vi "main(Test DQMH modules).vi"() -> ()   [LabVIEW 2018, in "Application.lvlib"] (continued)
        n2834 = Bundle By Name(cluster=w6304, "command"="Apps.WaitForEvent", "command data"=w6299) -> (w6303:T11)
        n2835 = Bundle By Name(cluster=w6304, "command"="MEAS.DMM dual read") -> (w6319:T11)
        n2836 = Bundle By Name(cluster=w6304, "command"="Apps.UI Update 1") -> (w6305:T11)
        n2837 = Build Array(w6319, w6318, w6303, w6305) -> (w6316:T11[])
        n2838 = Build Array (concatenate)(w6317, w6316) -> (w6315:T11[])
        n2839 = for {
          tunnel: w6315 -> [w6353] mode=indexing
          tunnel: w6310 -> [w6354]
          tunnel: [w6350] -> w6313 mode=indexing
          n2840 = Unbundle By Name(w6353) -> ("command"=w6352:string, "command data"=w6351:variant)
          n2841 = call "App enquece.vi"("command data"=w6351, "command"=w6352, "queue in"=w6354) -> ("error out"=w6350:errorcluster)  [unwired: 7 in, 1 out]
        }
        n2842 = Merge Errors(w6314, w6313) -> (w6312:errorcluster)
      }
      frame "Test DRV 6A" {
        w6361 = T11 {"command"="", "command data"=variant} ("element")
        w6355 = 6 ("DUT index(0-59)")
        w6387 = T11 {"command"="", "command data"=variant} ("element")
        n2843 = disable-structure shown="LOGGING==TRUE" {
          disable-tunnel: w6365 -> [w6403 _]
          frame condition #0 (active) {
            n2844 = Empty String/Path?(string/path=w6403) -> (empty?=w6406:bool)
            n2845 = Select(t="Quece timeout", s=w6406, f=w6403) -> (s? t:f=w6402:string)
            n2846 = call "string log (SubVI).vi"("Enum"=enum16{"Init", "Log", "Read"}."Log", "state Name"=w6402) -> ()  [unwired: 8 in, 2 out]
          }
          frame condition #1 {
          }
        }
        n2847 = Flush Queue(queue=w6366) -> (queue out=w6367:refnum<queue>)  [unwired: 1 in, 2 out]
        n2848 = Decrement(x=w6355) -> (x-1=w6359:i32)
        n2849 = Index Array(array=w6356, index=w6359) -> (element=w6357:refnum<vi>)
        n2850 = property class="ColBox"(reference=w6357, "Value"=u32 10000536 ("DRV 1")) -> ()  [unwired: 1 in, 2 out]
        n2851 = To Variant(anything=bool[] [FALSE, FALSE, FALSE, FALSE, FALSE, TRUE]) -> (Variant=w6384:variant)
        n2852 = To Variant(anything=T6."demux1_10_channel1" ("demux1_10(x6)_encode")) -> (Variant=w6388:variant)
        n2853 = To Variant(anything=T4."mux6_1_channel5_3" ("mux6_1(3wires)_encode")) -> (Variant=w6392:variant)
        n2854 = To Variant(anything=T5."mux10_1_channel1" ("mux10_1(x6)_encode")) -> (Variant=w6394:variant)
        n2855 = Bundle By Name(cluster=w6387, "command"="MEAS.mux10-1", "command data"=w6394) -> (w6382:T11)
        n2856 = Bundle By Name(cluster=w6387, "command"="MEAS.mux6_1", "command data"=w6392) -> (w6381:T11)
        n2857 = Bundle By Name(cluster=w6387, "command"="MEAS.demux1-10", "command data"=w6388) -> (w6380:T11)
        n2858 = Bundle By Name(cluster=w6387, "command"="MEAS.eMIC", "command data"=w6384) -> (w6379:T11)
        n2859 = Bundle By Name(cluster=w6387, "command"="MEAS.AllRelaysOFF") -> (w6383:T11)
        n2860 = Build Array(w6383, w6382, w6381, w6380, w6379) -> (w6374:T11[])
        n2861 = Bundle By Name(cluster=w6361, "command"="MEAS.requestAC", "command data"=w6355) -> (w6375:T11)
        n2862 = Bundle By Name(cluster=w6361, "command"="Apps.WaitForEvent", "command data"=w6355) -> (w6360:T11)
        n2863 = Bundle By Name(cluster=w6361, "command"="MEAS.DMM dual read") -> (w6376:T11)
        n2864 = Bundle By Name(cluster=w6361, "command"="Apps.UI Update 1") -> (w6362:T11)
        n2865 = Build Array(w6376, w6375, w6360, w6362) -> (w6373:T11[])
        n2866 = Build Array (concatenate)(w6374, w6373) -> (w6372:T11[])
        n2867 = for {
          tunnel: w6372 -> [w6410] mode=indexing
          tunnel: w6367 -> [w6411]
          tunnel: [w6407] -> w6370 mode=indexing
          n2868 = Unbundle By Name(w6410) -> ("command"=w6409:string, "command data"=w6408:variant)
          n2869 = call "App enquece.vi"("command data"=w6408, "command"=w6409, "queue in"=w6411) -> ("error out"=w6407:errorcluster)  [unwired: 7 in, 1 out]
        }
        n2870 = Merge Errors(w6371, w6370) -> (w6369:errorcluster)
      }
      frame "Test DRV 7A" {
        w6418 = T11 {"command"="", "command data"=variant} ("element")
        w6412 = 7 ("DUT index(0-59)")
        w6444 = T11 {"command"="", "command data"=variant} ("element")
        n2871 = disable-structure shown="LOGGING==TRUE" {
          disable-tunnel: w6422 -> [w6460 _]
          frame condition #0 (active) {
            n2872 = Empty String/Path?(string/path=w6460) -> (empty?=w6463:bool)
            n2873 = Select(t="Quece timeout", s=w6463, f=w6460) -> (s? t:f=w6459:string)
            n2874 = call "string log (SubVI).vi"("Enum"=enum16{"Init", "Log", "Read"}."Log", "state Name"=w6459) -> ()  [unwired: 8 in, 2 out]
          }
          frame condition #1 {
          }
        }
        n2875 = Flush Queue(queue=w6423) -> (queue out=w6424:refnum<queue>)  [unwired: 1 in, 2 out]
        n2876 = Decrement(x=w6412) -> (x-1=w6416:i32)
        n2877 = Index Array(array=w6413, index=w6416) -> (element=w6414:refnum<vi>)
        n2878 = property class="ColBox"(reference=w6414, "Value"=u32 10000536 ("DRV 1")) -> ()  [unwired: 1 in, 2 out]
        n2879 = To Variant(anything=bool[] [TRUE, FALSE, FALSE, FALSE, FALSE, FALSE]) -> (Variant=w6441:variant)
        n2880 = To Variant(anything=T6."demux1_10_channel2" ("demux1_10(x6)_encode")) -> (Variant=w6445:variant)
        n2881 = To Variant(anything=T4."mux6_1_channel1_3" ("mux6_1(3wires)_encode")) -> (Variant=w6449:variant)
        n2882 = To Variant(anything=T5."mux10_1_channel2" ("mux10_1(x6)_encode")) -> (Variant=w6451:variant)
        n2883 = Bundle By Name(cluster=w6444, "command"="MEAS.mux10-1", "command data"=w6451) -> (w6439:T11)
        n2884 = Bundle By Name(cluster=w6444, "command"="MEAS.mux6_1", "command data"=w6449) -> (w6438:T11)
        n2885 = Bundle By Name(cluster=w6444, "command"="MEAS.demux1-10", "command data"=w6445) -> (w6437:T11)
        n2886 = Bundle By Name(cluster=w6444, "command"="MEAS.eMIC", "command data"=w6441) -> (w6436:T11)
        n2887 = Bundle By Name(cluster=w6444, "command"="MEAS.AllRelaysOFF") -> (w6440:T11)
        n2888 = Build Array(w6440, w6439, w6438, w6437, w6436) -> (w6431:T11[])
        n2889 = Bundle By Name(cluster=w6418, "command"="MEAS.requestAC", "command data"=w6412) -> (w6432:T11)
        n2890 = Bundle By Name(cluster=w6418, "command"="Apps.WaitForEvent", "command data"=w6412) -> (w6417:T11)
        n2891 = Bundle By Name(cluster=w6418, "command"="MEAS.DMM dual read") -> (w6433:T11)
        n2892 = Bundle By Name(cluster=w6418, "command"="Apps.UI Update 1") -> (w6419:T11)
        n2893 = Build Array(w6433, w6432, w6417, w6419) -> (w6430:T11[])
        n2894 = Build Array (concatenate)(w6431, w6430) -> (w6429:T11[])
        n2895 = for {
          tunnel: w6429 -> [w6467] mode=indexing
          tunnel: w6424 -> [w6468]
          tunnel: [w6464] -> w6427 mode=indexing
          n2896 = Unbundle By Name(w6467) -> ("command"=w6466:string, "command data"=w6465:variant)
          n2897 = call "App enquece.vi"("command data"=w6465, "command"=w6466, "queue in"=w6468) -> ("error out"=w6464:errorcluster)  [unwired: 7 in, 1 out]
        }
        n2898 = Merge Errors(w6428, w6427) -> (w6426:errorcluster)
      }
      frame "Test DRV 8A" {
        w6475 = T11 {"command"="", "command data"=variant} ("element")
        w6469 = 8 ("DUT index(0-59)")
        w6501 = T11 {"command"="", "command data"=variant} ("element")
        n2899 = disable-structure shown="LOGGING==TRUE" {
          disable-tunnel: w6479 -> [w6517 _]
          frame condition #0 (active) {
            n2900 = Empty String/Path?(string/path=w6517) -> (empty?=w6520:bool)
            n2901 = Select(t="Quece timeout", s=w6520, f=w6517) -> (s? t:f=w6516:string)
            n2902 = call "string log (SubVI).vi"("Enum"=enum16{"Init", "Log", "Read"}."Log", "state Name"=w6516) -> ()  [unwired: 8 in, 2 out]
          }
          frame condition #1 {
          }
        }
        n2903 = Flush Queue(queue=w6480) -> (queue out=w6481:refnum<queue>)  [unwired: 1 in, 2 out]
        n2904 = Decrement(x=w6469) -> (x-1=w6473:i32)
        n2905 = Index Array(array=w6470, index=w6473) -> (element=w6471:refnum<vi>)
        n2906 = property class="ColBox"(reference=w6471, "Value"=u32 10000536 ("DRV 1")) -> ()  [unwired: 1 in, 2 out]
        n2907 = To Variant(anything=bool[] [FALSE, TRUE, FALSE, FALSE, FALSE, FALSE]) -> (Variant=w6498:variant)
        n2908 = To Variant(anything=T6."demux1_10_channel2" ("demux1_10(x6)_encode")) -> (Variant=w6502:variant)
        n2909 = To Variant(anything=T4."mux6_1_channel2_3" ("mux6_1(3wires)_encode")) -> (Variant=w6506:variant)
        n2910 = To Variant(anything=T5."mux10_1_channel2" ("mux10_1(x6)_encode")) -> (Variant=w6508:variant)
        n2911 = Bundle By Name(cluster=w6501, "command"="MEAS.mux10-1", "command data"=w6508) -> (w6496:T11)
        n2912 = Bundle By Name(cluster=w6501, "command"="MEAS.mux6_1", "command data"=w6506) -> (w6495:T11)
        n2913 = Bundle By Name(cluster=w6501, "command"="MEAS.demux1-10", "command data"=w6502) -> (w6494:T11)
        n2914 = Bundle By Name(cluster=w6501, "command"="MEAS.eMIC", "command data"=w6498) -> (w6493:T11)
        n2915 = Bundle By Name(cluster=w6501, "command"="MEAS.AllRelaysOFF") -> (w6497:T11)
        n2916 = Build Array(w6497, w6496, w6495, w6494, w6493) -> (w6488:T11[])
        n2917 = Bundle By Name(cluster=w6475, "command"="MEAS.requestAC", "command data"=w6469) -> (w6489:T11)
        n2918 = Bundle By Name(cluster=w6475, "command"="Apps.WaitForEvent", "command data"=w6469) -> (w6474:T11)
        n2919 = Bundle By Name(cluster=w6475, "command"="MEAS.DMM dual read") -> (w6490:T11)
        n2920 = Bundle By Name(cluster=w6475, "command"="Apps.UI Update 1") -> (w6476:T11)
        n2921 = Build Array(w6490, w6489, w6474, w6476) -> (w6487:T11[])
        n2922 = Build Array (concatenate)(w6488, w6487) -> (w6486:T11[])
        n2923 = for {
          tunnel: w6486 -> [w6524] mode=indexing
          tunnel: w6481 -> [w6525]
          tunnel: [w6521] -> w6484 mode=indexing
          n2924 = Unbundle By Name(w6524) -> ("command"=w6523:string, "command data"=w6522:variant)
          n2925 = call "App enquece.vi"("command data"=w6522, "command"=w6523, "queue in"=w6525) -> ("error out"=w6521:errorcluster)  [unwired: 7 in, 1 out]
        }
        n2926 = Merge Errors(w6485, w6484) -> (w6483:errorcluster)
      }
      frame "Test DRV 9A" {
        w6532 = T11 {"command"="", "command data"=variant} ("element")
        w6526 = 9 ("DUT index(0-59)")
        w6558 = T11 {"command"="", "command data"=variant} ("element")
        n2927 = disable-structure shown="LOGGING==TRUE" {
          disable-tunnel: w6536 -> [w6574 _]
          frame condition #0 (active) {
            n2928 = Empty String/Path?(string/path=w6574) -> (empty?=w6577:bool)
            n2929 = Select(t="Quece timeout", s=w6577, f=w6574) -> (s? t:f=w6573:string)
            n2930 = call "string log (SubVI).vi"("Enum"=enum16{"Init", "Log", "Read"}."Log", "state Name"=w6573) -> ()  [unwired: 8 in, 2 out]
          }
          frame condition #1 {
          }
        }
        n2931 = Flush Queue(queue=w6537) -> (queue out=w6538:refnum<queue>)  [unwired: 1 in, 2 out]
        n2932 = Decrement(x=w6526) -> (x-1=w6530:i32)
        n2933 = Index Array(array=w6527, index=w6530) -> (element=w6528:refnum<vi>)
        n2934 = property class="ColBox"(reference=w6528, "Value"=u32 10000536 ("DRV 1")) -> ()  [unwired: 1 in, 2 out]
        n2935 = To Variant(anything=bool[] [FALSE, FALSE, TRUE, FALSE, FALSE, FALSE]) -> (Variant=w6555:variant)
        n2936 = To Variant(anything=T6."demux1_10_channel2" ("demux1_10(x6)_encode")) -> (Variant=w6559:variant)
        n2937 = To Variant(anything=T4."mux6_1_channel3_3" ("mux6_1(3wires)_encode")) -> (Variant=w6563:variant)
        n2938 = To Variant(anything=T5."mux10_1_channel2" ("mux10_1(x6)_encode")) -> (Variant=w6565:variant)
        n2939 = Bundle By Name(cluster=w6558, "command"="MEAS.mux10-1", "command data"=w6565) -> (w6553:T11)
        n2940 = Bundle By Name(cluster=w6558, "command"="MEAS.mux6_1", "command data"=w6563) -> (w6552:T11)
        n2941 = Bundle By Name(cluster=w6558, "command"="MEAS.demux1-10", "command data"=w6559) -> (w6551:T11)
        n2942 = Bundle By Name(cluster=w6558, "command"="MEAS.eMIC", "command data"=w6555) -> (w6550:T11)
        n2943 = Bundle By Name(cluster=w6558, "command"="MEAS.AllRelaysOFF") -> (w6554:T11)
        n2944 = Build Array(w6554, w6553, w6552, w6551, w6550) -> (w6545:T11[])
        n2945 = Bundle By Name(cluster=w6532, "command"="MEAS.requestAC", "command data"=w6526) -> (w6546:T11)
        n2946 = Bundle By Name(cluster=w6532, "command"="Apps.WaitForEvent", "command data"=w6526) -> (w6531:T11)
        n2947 = Bundle By Name(cluster=w6532, "command"="MEAS.DMM dual read") -> (w6547:T11)
        n2948 = Bundle By Name(cluster=w6532, "command"="Apps.UI Update 1") -> (w6533:T11)
        n2949 = Build Array(w6547, w6546, w6531, w6533) -> (w6544:T11[])
        n2950 = Build Array (concatenate)(w6545, w6544) -> (w6543:T11[])
        n2951 = for {
          tunnel: w6543 -> [w6581] mode=indexing
          tunnel: w6538 -> [w6582]
          tunnel: [w6578] -> w6541 mode=indexing
          n2952 = Unbundle By Name(w6581) -> ("command"=w6580:string, "command data"=w6579:variant)
          n2953 = call "App enquece.vi"("command data"=w6579, "command"=w6580, "queue in"=w6582) -> ("error out"=w6578:errorcluster)  [unwired: 7 in, 1 out]
        }
        n2954 = Merge Errors(w6542, w6541) -> (w6540:errorcluster)
      }
      frame "Test DRV 10A" {
        w6589 = T11 {"command"="", "command data"=variant} ("element")
        w6583 = 10 ("DUT index(0-59)")
        w6615 = T11 {"command"="", "command data"=variant} ("element")
        n2955 = disable-structure shown="LOGGING==TRUE" {
          disable-tunnel: w6593 -> [w6631 _]
          frame condition #0 (active) {
            n2956 = Empty String/Path?(string/path=w6631) -> (empty?=w6634:bool)
            n2957 = Select(t="Quece timeout", s=w6634, f=w6631) -> (s? t:f=w6630:string)
            n2958 = call "string log (SubVI).vi"("Enum"=enum16{"Init", "Log", "Read"}."Log", "state Name"=w6630) -> ()  [unwired: 8 in, 2 out]
          }
          frame condition #1 {
          }
        }
        n2959 = Flush Queue(queue=w6594) -> (queue out=w6595:refnum<queue>)  [unwired: 1 in, 2 out]
        n2960 = Decrement(x=w6583) -> (x-1=w6587:i32)
        n2961 = Index Array(array=w6584, index=w6587) -> (element=w6585:refnum<vi>)
        n2962 = property class="ColBox"(reference=w6585, "Value"=u32 10000536 ("DRV 1")) -> ()  [unwired: 1 in, 2 out]
        n2963 = To Variant(anything=bool[] [FALSE, FALSE, FALSE, TRUE, FALSE, FALSE]) -> (Variant=w6612:variant)
        n2964 = To Variant(anything=T6."demux1_10_channel2" ("demux1_10(x6)_encode")) -> (Variant=w6616:variant)
        n2965 = To Variant(anything=T4."mux6_1_channel4_3" ("mux6_1(3wires)_encode")) -> (Variant=w6620:variant)
        n2966 = To Variant(anything=T5."mux10_1_channel2" ("mux10_1(x6)_encode")) -> (Variant=w6622:variant)
        n2967 = Bundle By Name(cluster=w6615, "command"="MEAS.mux10-1", "command data"=w6622) -> (w6610:T11)
        n2968 = Bundle By Name(cluster=w6615, "command"="MEAS.mux6_1", "command data"=w6620) -> (w6609:T11)
        n2969 = Bundle By Name(cluster=w6615, "command"="MEAS.demux1-10", "command data"=w6616) -> (w6608:T11)
        n2970 = Bundle By Name(cluster=w6615, "command"="MEAS.eMIC", "command data"=w6612) -> (w6607:T11)
        n2971 = Bundle By Name(cluster=w6615, "command"="MEAS.AllRelaysOFF") -> (w6611:T11)
        n2972 = Build Array(w6611, w6610, w6609, w6608, w6607) -> (w6602:T11[])
        n2973 = Bundle By Name(cluster=w6589, "command"="MEAS.requestAC", "command data"=w6583) -> (w6603:T11)
        n2974 = Bundle By Name(cluster=w6589, "command"="Apps.WaitForEvent", "command data"=w6583) -> (w6588:T11)
        n2975 = Bundle By Name(cluster=w6589, "command"="MEAS.DMM dual read") -> (w6604:T11)
        n2976 = Bundle By Name(cluster=w6589, "command"="Apps.UI Update 1") -> (w6590:T11)
        n2977 = Build Array(w6604, w6603, w6588, w6590) -> (w6601:T11[])
        n2978 = Build Array (concatenate)(w6602, w6601) -> (w6600:T11[])
        n2979 = for {
          tunnel: w6600 -> [w6638] mode=indexing
          tunnel: w6595 -> [w6639]
          tunnel: [w6635] -> w6598 mode=indexing
          n2980 = Unbundle By Name(w6638) -> ("command"=w6637:string, "command data"=w6636:variant)
          n2981 = call "App enquece.vi"("command data"=w6636, "command"=w6637, "queue in"=w6639) -> ("error out"=w6635:errorcluster)  [unwired: 7 in, 1 out]
        }
        n2982 = Merge Errors(w6599, w6598) -> (w6597:errorcluster)
      }
      frame "Test DRV 11A" {
        w6646 = T11 {"command"="", "command data"=variant} ("element")
        w6640 = 11 ("DUT index(0-59)")
        w6672 = T11 {"command"="", "command data"=variant} ("element")
        n2983 = disable-structure shown="LOGGING==TRUE" {
          disable-tunnel: w6650 -> [w6688 _]
          frame condition #0 (active) {
            n2984 = Empty String/Path?(string/path=w6688) -> (empty?=w6691:bool)
            n2985 = Select(t="Quece timeout", s=w6691, f=w6688) -> (s? t:f=w6687:string)
            n2986 = call "string log (SubVI).vi"("Enum"=enum16{"Init", "Log", "Read"}."Log", "state Name"=w6687) -> ()  [unwired: 8 in, 2 out]
          }
          frame condition #1 {
          }
        }
        n2987 = Flush Queue(queue=w6651) -> (queue out=w6652:refnum<queue>)  [unwired: 1 in, 2 out]
        n2988 = Decrement(x=w6640) -> (x-1=w6644:i32)
        n2989 = Index Array(array=w6641, index=w6644) -> (element=w6642:refnum<vi>)
        n2990 = property class="ColBox"(reference=w6642, "Value"=u32 10000536 ("DRV 1")) -> ()  [unwired: 1 in, 2 out]
        n2991 = To Variant(anything=bool[] [FALSE, FALSE, FALSE, FALSE, TRUE, FALSE]) -> (Variant=w6669:variant)
        n2992 = To Variant(anything=T6."demux1_10_channel2" ("demux1_10(x6)_encode")) -> (Variant=w6673:variant)
        n2993 = To Variant(anything=T4."mux6_1_channel5_3" ("mux6_1(3wires)_encode")) -> (Variant=w6677:variant)
        n2994 = To Variant(anything=T5."mux10_1_channel2" ("mux10_1(x6)_encode")) -> (Variant=w6679:variant)
        n2995 = Bundle By Name(cluster=w6672, "command"="MEAS.mux10-1", "command data"=w6679) -> (w6667:T11)
        n2996 = Bundle By Name(cluster=w6672, "command"="MEAS.mux6_1", "command data"=w6677) -> (w6666:T11)
        n2997 = Bundle By Name(cluster=w6672, "command"="MEAS.demux1-10", "command data"=w6673) -> (w6665:T11)
        n2998 = Bundle By Name(cluster=w6672, "command"="MEAS.eMIC", "command data"=w6669) -> (w6664:T11)
        n2999 = Bundle By Name(cluster=w6672, "command"="MEAS.AllRelaysOFF") -> (w6668:T11)
        n3000 = Build Array(w6668, w6667, w6666, w6665, w6664) -> (w6659:T11[])
        n3001 = Bundle By Name(cluster=w6646, "command"="MEAS.requestAC", "command data"=w6640) -> (w6660:T11)
        n3002 = Bundle By Name(cluster=w6646, "command"="Apps.WaitForEvent", "command data"=w6640) -> (w6645:T11)
        n3003 = Bundle By Name(cluster=w6646, "command"="MEAS.DMM dual read") -> (w6661:T11)
        n3004 = Bundle By Name(cluster=w6646, "command"="Apps.UI Update 1") -> (w6647:T11)
        n3005 = Build Array(w6661, w6660, w6645, w6647) -> (w6658:T11[])
        n3006 = Build Array (concatenate)(w6659, w6658) -> (w6657:T11[])
        n3007 = for {
          tunnel: w6657 -> [w6695] mode=indexing
          tunnel: w6652 -> [w6696]
          tunnel: [w6692] -> w6655 mode=indexing
          n3008 = Unbundle By Name(w6695) -> ("command"=w6694:string, "command data"=w6693:variant)
          n3009 = call "App enquece.vi"("command data"=w6693, "command"=w6694, "queue in"=w6696) -> ("error out"=w6692:errorcluster)  [unwired: 7 in, 1 out]
        }
        n3010 = Merge Errors(w6656, w6655) -> (w6654:errorcluster)
      }
      frame "Test DRV 12A" {
        w6703 = T11 {"command"="", "command data"=variant} ("element")
        w6697 = 12 ("DUT index(0-59)")
        w6729 = T11 {"command"="", "command data"=variant} ("element")
        n3011 = disable-structure shown="LOGGING==TRUE" {
          disable-tunnel: w6707 -> [w6745 _]
          frame condition #0 (active) {
            n3012 = Empty String/Path?(string/path=w6745) -> (empty?=w6748:bool)
            n3013 = Select(t="Quece timeout", s=w6748, f=w6745) -> (s? t:f=w6744:string)
            n3014 = call "string log (SubVI).vi"("Enum"=enum16{"Init", "Log", "Read"}."Log", "state Name"=w6744) -> ()  [unwired: 8 in, 2 out]
          }
          frame condition #1 {
          }
        }
        n3015 = Flush Queue(queue=w6708) -> (queue out=w6709:refnum<queue>)  [unwired: 1 in, 2 out]
        n3016 = Decrement(x=w6697) -> (x-1=w6701:i32)
        n3017 = Index Array(array=w6698, index=w6701) -> (element=w6699:refnum<vi>)
        n3018 = property class="ColBox"(reference=w6699, "Value"=u32 10000536 ("DRV 1")) -> ()  [unwired: 1 in, 2 out]
        n3019 = To Variant(anything=bool[] [FALSE, FALSE, FALSE, FALSE, FALSE, TRUE]) -> (Variant=w6726:variant)
        n3020 = To Variant(anything=T6."demux1_10_channel2" ("demux1_10(x6)_encode")) -> (Variant=w6730:variant)
        n3021 = To Variant(anything=T4."mux6_1_channel6_3" ("mux6_1(3wires)_encode")) -> (Variant=w6734:variant)
        n3022 = To Variant(anything=T5."mux10_1_channel2" ("mux10_1(x6)_encode")) -> (Variant=w6736:variant)
        n3023 = Bundle By Name(cluster=w6729, "command"="MEAS.mux10-1", "command data"=w6736) -> (w6724:T11)
        n3024 = Bundle By Name(cluster=w6729, "command"="MEAS.mux6_1", "command data"=w6734) -> (w6723:T11)
        n3025 = Bundle By Name(cluster=w6729, "command"="MEAS.demux1-10", "command data"=w6730) -> (w6722:T11)
        n3026 = Bundle By Name(cluster=w6729, "command"="MEAS.eMIC", "command data"=w6726) -> (w6721:T11)
        n3027 = Bundle By Name(cluster=w6729, "command"="MEAS.AllRelaysOFF") -> (w6725:T11)
        n3028 = Build Array(w6725, w6724, w6723, w6722, w6721) -> (w6716:T11[])
        n3029 = Bundle By Name(cluster=w6703, "command"="MEAS.requestAC", "command data"=w6697) -> (w6717:T11)
        n3030 = Bundle By Name(cluster=w6703, "command"="Apps.WaitForEvent", "command data"=w6697) -> (w6702:T11)
        n3031 = Bundle By Name(cluster=w6703, "command"="MEAS.DMM dual read") -> (w6718:T11)
        n3032 = Bundle By Name(cluster=w6703, "command"="Apps.UI Update 1") -> (w6704:T11)
        n3033 = Build Array(w6718, w6717, w6702, w6704) -> (w6715:T11[])
        n3034 = Build Array (concatenate)(w6716, w6715) -> (w6714:T11[])
        n3035 = for {
          tunnel: w6714 -> [w6752] mode=indexing
          tunnel: w6709 -> [w6753]
          tunnel: [w6749] -> w6712 mode=indexing
          n3036 = Unbundle By Name(w6752) -> ("command"=w6751:string, "command data"=w6750:variant)
          n3037 = call "App enquece.vi"("command data"=w6750, "command"=w6751, "queue in"=w6753) -> ("error out"=w6749:errorcluster)  [unwired: 7 in, 1 out]
        }
        n3038 = Merge Errors(w6713, w6712) -> (w6711:errorcluster)
      }
      frame "Test DRV 13A" {
        w6760 = T11 {"command"="", "command data"=variant} ("element")
        w6755 = 13 ("DUT index(0-59)")
        w6786 = T11 {"command"="", "command data"=variant} ("element")
        n3039 = disable-structure shown="LOGGING==TRUE" {
          disable-tunnel: w6764 -> [w6802 _]
          frame condition #0 (active) {
            n3040 = Empty String/Path?(string/path=w6802) -> (empty?=w6805:bool)
            n3041 = Select(t="Quece timeout", s=w6805, f=w6802) -> (s? t:f=w6801:string)
            n3042 = call "string log (SubVI).vi"("Enum"=enum16{"Init", "Log", "Read"}."Log", "state Name"=w6801) -> ()  [unwired: 8 in, 2 out]
          }
          frame condition #1 {
          }
        }
        n3043 = Flush Queue(queue=w6765) -> (queue out=w6766:refnum<queue>)  [unwired: 1 in, 2 out]
        n3044 = Decrement(x=w6755) -> (x-1=w6758:i32)
        n3045 = Index Array(array=w6754, index=w6758) -> (element=w6756:refnum<vi>)
        n3046 = property class="ColBox"(reference=w6756, "Value"=u32 10000536 ("DRV 1")) -> ()  [unwired: 1 in, 2 out]
        n3047 = To Variant(anything=bool[] [TRUE, FALSE, FALSE, FALSE, FALSE, FALSE]) -> (Variant=w6783:variant)
        n3048 = To Variant(anything=T6."demux1_10_channel3" ("demux1_10(x6)_encode")) -> (Variant=w6787:variant)
        n3049 = To Variant(anything=T4."mux6_1_channel1_3" ("mux6_1(3wires)_encode")) -> (Variant=w6791:variant)
        n3050 = To Variant(anything=T5."mux10_1_channel3" ("mux10_1(x6)_encode")) -> (Variant=w6793:variant)
        n3051 = Bundle By Name(cluster=w6786, "command"="MEAS.mux10-1", "command data"=w6793) -> (w6781:T11)
        n3052 = Bundle By Name(cluster=w6786, "command"="MEAS.mux6_1", "command data"=w6791) -> (w6780:T11)
        n3053 = Bundle By Name(cluster=w6786, "command"="MEAS.demux1-10", "command data"=w6787) -> (w6779:T11)
        n3054 = Bundle By Name(cluster=w6786, "command"="MEAS.eMIC", "command data"=w6783) -> (w6778:T11)
        n3055 = Bundle By Name(cluster=w6786, "command"="MEAS.AllRelaysOFF") -> (w6782:T11)
        n3056 = Build Array(w6782, w6781, w6780, w6779, w6778) -> (w6773:T11[])
        n3057 = Bundle By Name(cluster=w6760, "command"="MEAS.requestAC", "command data"=w6755) -> (w6774:T11)
        n3058 = Bundle By Name(cluster=w6760, "command"="Apps.WaitForEvent", "command data"=w6755) -> (w6759:T11)
        n3059 = Bundle By Name(cluster=w6760, "command"="MEAS.DMM dual read") -> (w6775:T11)
        n3060 = Bundle By Name(cluster=w6760, "command"="Apps.UI Update 1") -> (w6761:T11)
        n3061 = Build Array(w6775, w6774, w6759, w6761) -> (w6772:T11[])
        n3062 = Build Array (concatenate)(w6773, w6772) -> (w6771:T11[])
        n3063 = for {
          tunnel: w6771 -> [w6809] mode=indexing
          tunnel: w6766 -> [w6810]
          tunnel: [w6806] -> w6769 mode=indexing
          n3064 = Unbundle By Name(w6809) -> ("command"=w6808:string, "command data"=w6807:variant)
          n3065 = call "App enquece.vi"("command data"=w6807, "command"=w6808, "queue in"=w6810) -> ("error out"=w6806:errorcluster)  [unwired: 7 in, 1 out]
        }
        n3066 = Merge Errors(w6770, w6769) -> (w6768:errorcluster)
      }
      frame "Test DRV 14A" {
        w6817 = T11 {"command"="", "command data"=variant} ("element")
        w6812 = 14 ("DUT index(0-59)")
        w6843 = T11 {"command"="", "command data"=variant} ("element")
        n3067 = disable-structure shown="LOGGING==TRUE" {
          disable-tunnel: w6821 -> [w6859 _]
          frame condition #0 (active) {
            n3068 = Empty String/Path?(string/path=w6859) -> (empty?=w6862:bool)
            n3069 = Select(t="Quece timeout", s=w6862, f=w6859) -> (s? t:f=w6858:string)
            n3070 = call "string log (SubVI).vi"("Enum"=enum16{"Init", "Log", "Read"}."Log", "state Name"=w6858) -> ()  [unwired: 8 in, 2 out]
          }
          frame condition #1 {
          }
        }
        n3071 = Flush Queue(queue=w6822) -> (queue out=w6823:refnum<queue>)  [unwired: 1 in, 2 out]
        n3072 = Decrement(x=w6812) -> (x-1=w6815:i32)
        n3073 = Index Array(array=w6811, index=w6815) -> (element=w6813:refnum<vi>)
        n3074 = property class="ColBox"(reference=w6813, "Value"=u32 10000536 ("DRV 1")) -> ()  [unwired: 1 in, 2 out]
        n3075 = To Variant(anything=bool[] [FALSE, TRUE, FALSE, FALSE, FALSE, FALSE]) -> (Variant=w6840:variant)
        n3076 = To Variant(anything=T6."demux1_10_channel3" ("demux1_10(x6)_encode")) -> (Variant=w6844:variant)
        n3077 = To Variant(anything=T4."mux6_1_channel2_3" ("mux6_1(3wires)_encode")) -> (Variant=w6848:variant)
        n3078 = To Variant(anything=T5."mux10_1_channel3" ("mux10_1(x6)_encode")) -> (Variant=w6850:variant)
        n3079 = Bundle By Name(cluster=w6843, "command"="MEAS.mux10-1", "command data"=w6850) -> (w6838:T11)
        n3080 = Bundle By Name(cluster=w6843, "command"="MEAS.mux6_1", "command data"=w6848) -> (w6837:T11)
        n3081 = Bundle By Name(cluster=w6843, "command"="MEAS.demux1-10", "command data"=w6844) -> (w6836:T11)
        n3082 = Bundle By Name(cluster=w6843, "command"="MEAS.eMIC", "command data"=w6840) -> (w6835:T11)
        n3083 = Bundle By Name(cluster=w6843, "command"="MEAS.AllRelaysOFF") -> (w6839:T11)
        n3084 = Build Array(w6839, w6838, w6837, w6836, w6835) -> (w6830:T11[])
        n3085 = Bundle By Name(cluster=w6817, "command"="MEAS.requestAC", "command data"=w6812) -> (w6831:T11)
        n3086 = Bundle By Name(cluster=w6817, "command"="Apps.WaitForEvent", "command data"=w6812) -> (w6816:T11)
        n3087 = Bundle By Name(cluster=w6817, "command"="MEAS.DMM dual read") -> (w6832:T11)
        n3088 = Bundle By Name(cluster=w6817, "command"="Apps.UI Update 1") -> (w6818:T11)
        n3089 = Build Array(w6832, w6831, w6816, w6818) -> (w6829:T11[])
        n3090 = Build Array (concatenate)(w6830, w6829) -> (w6828:T11[])
        n3091 = for {
          tunnel: w6828 -> [w6866] mode=indexing
          tunnel: w6823 -> [w6867]
          tunnel: [w6863] -> w6826 mode=indexing
          n3092 = Unbundle By Name(w6866) -> ("command"=w6865:string, "command data"=w6864:variant)
          n3093 = call "App enquece.vi"("command data"=w6864, "command"=w6865, "queue in"=w6867) -> ("error out"=w6863:errorcluster)  [unwired: 7 in, 1 out]
        }
        n3094 = Merge Errors(w6827, w6826) -> (w6825:errorcluster)
      }
      frame "Test DRV 15A" {
        w6875 = T11 {"command"="", "command data"=variant} ("element")
        w6869 = 15 ("DUT index(0-59)")
        w6901 = T11 {"command"="", "command data"=variant} ("element")
        n3095 = disable-structure shown="LOGGING==TRUE" {
          disable-tunnel: w6879 -> [w6916 _]
          frame condition #0 (active) {
            n3096 = Empty String/Path?(string/path=w6916) -> (empty?=w6919:bool)
            n3097 = Select(t="Quece timeout", s=w6919, f=w6916) -> (s? t:f=w6915:string)
            n3098 = call "string log (SubVI).vi"("Enum"=enum16{"Init", "Log", "Read"}."Log", "state Name"=w6915) -> ()  [unwired: 8 in, 2 out]
          }
          frame condition #1 {
          }
        }
        n3099 = Flush Queue(queue=w6880) -> (queue out=w6881:refnum<queue>)  [unwired: 1 in, 2 out]
        n3100 = Decrement(x=w6869) -> (x-1=w6872:i32)
        n3101 = Index Array(array=w6868, index=w6872) -> (element=w6870:refnum<vi>)
        n3102 = property class="ColBox"(reference=w6870, "Value"=u32 10000536 ("DRV 1")) -> ()  [unwired: 1 in, 2 out]
        n3103 = To Variant(anything=bool[] [FALSE, FALSE, TRUE, FALSE, FALSE, FALSE]) -> (Variant=w6898:variant)
        n3104 = To Variant(anything=T6."demux1_10_channel3" ("demux1_10(x6)_encode")) -> (Variant=w6902:variant)
        n3105 = To Variant(anything=T4."mux6_1_channel3_3" ("mux6_1(3wires)_encode")) -> (Variant=w6905:variant)
        n3106 = To Variant(anything=T5."mux10_1_channel3" ("mux10_1(x6)_encode")) -> (Variant=w6907:variant)
        n3107 = Bundle By Name(cluster=w6901, "command"="MEAS.mux10-1", "command data"=w6907) -> (w6896:T11)
        n3108 = Bundle By Name(cluster=w6901, "command"="MEAS.mux6_1", "command data"=w6905) -> (w6895:T11)
        n3109 = Bundle By Name(cluster=w6901, "command"="MEAS.demux1-10", "command data"=w6902) -> (w6894:T11)
        n3110 = Bundle By Name(cluster=w6901, "command"="MEAS.eMIC", "command data"=w6898) -> (w6893:T11)
        n3111 = Bundle By Name(cluster=w6901, "command"="MEAS.AllRelaysOFF") -> (w6897:T11)
        n3112 = Build Array(w6897, w6896, w6895, w6894, w6893) -> (w6888:T11[])
        n3113 = Bundle By Name(cluster=w6875, "command"="MEAS.requestAC", "command data"=w6869) -> (w6889:T11)
        n3114 = Bundle By Name(cluster=w6875, "command"="Apps.WaitForEvent", "command data"=w6869) -> (w6874:T11)
        n3115 = Bundle By Name(cluster=w6875, "command"="MEAS.DMM dual read") -> (w6890:T11)
        n3116 = Bundle By Name(cluster=w6875, "command"="Apps.UI Update 1") -> (w6876:T11)
        n3117 = Build Array(w6890, w6889, w6874, w6876) -> (w6887:T11[])
        n3118 = Build Array (concatenate)(w6888, w6887) -> (w6886:T11[])
        n3119 = for {
          tunnel: w6886 -> [w6923] mode=indexing
          tunnel: w6881 -> [w6924]
          tunnel: [w6920] -> w6884 mode=indexing
          n3120 = Unbundle By Name(w6923) -> ("command"=w6922:string, "command data"=w6921:variant)
          n3121 = call "App enquece.vi"("command data"=w6921, "command"=w6922, "queue in"=w6924) -> ("error out"=w6920:errorcluster)  [unwired: 7 in, 1 out]
        }
        n3122 = Merge Errors(w6885, w6884) -> (w6883:errorcluster)
      }
      frame "Test DRV 16A" {
        w6932 = T11 {"command"="", "command data"=variant} ("element")
        w6926 = 16 ("DUT index(0-59)")
        w6958 = T11 {"command"="", "command data"=variant} ("element")
        n3123 = disable-structure shown="LOGGING==TRUE" {
          disable-tunnel: w6936 -> [w6973 _]
          frame condition #0 (active) {
            n3124 = Empty String/Path?(string/path=w6973) -> (empty?=w6976:bool)
            n3125 = Select(t="Quece timeout", s=w6976, f=w6973) -> (s? t:f=w6972:string)
            n3126 = call "string log (SubVI).vi"("Enum"=enum16{"Init", "Log", "Read"}."Log", "state Name"=w6972) -> ()  [unwired: 8 in, 2 out]
          }
          frame condition #1 {
          }
        }
        n3127 = Flush Queue(queue=w6937) -> (queue out=w6938:refnum<queue>)  [unwired: 1 in, 2 out]
        n3128 = Decrement(x=w6926) -> (x-1=w6929:i32)
        n3129 = Index Array(array=w6925, index=w6929) -> (element=w6927:refnum<vi>)
        n3130 = property class="ColBox"(reference=w6927, "Value"=u32 10000536 ("DRV 1")) -> ()  [unwired: 1 in, 2 out]
        n3131 = To Variant(anything=bool[] [FALSE, FALSE, FALSE, TRUE, FALSE, FALSE]) -> (Variant=w6955:variant)
        n3132 = To Variant(anything=T6."demux1_10_channel3" ("demux1_10(x6)_encode")) -> (Variant=w6959:variant)
        n3133 = To Variant(anything=T4."mux6_1_channel4_3" ("mux6_1(3wires)_encode")) -> (Variant=w6962:variant)
        n3134 = To Variant(anything=T5."mux10_1_channel3" ("mux10_1(x6)_encode")) -> (Variant=w6964:variant)
        n3135 = Bundle By Name(cluster=w6958, "command"="MEAS.mux10-1", "command data"=w6964) -> (w6953:T11)
        n3136 = Bundle By Name(cluster=w6958, "command"="MEAS.mux6_1", "command data"=w6962) -> (w6952:T11)
        n3137 = Bundle By Name(cluster=w6958, "command"="MEAS.demux1-10", "command data"=w6959) -> (w6951:T11)
        n3138 = Bundle By Name(cluster=w6958, "command"="MEAS.eMIC", "command data"=w6955) -> (w6950:T11)
        n3139 = Bundle By Name(cluster=w6958, "command"="MEAS.AllRelaysOFF") -> (w6954:T11)
        n3140 = Build Array(w6954, w6953, w6952, w6951, w6950) -> (w6945:T11[])
        n3141 = Bundle By Name(cluster=w6932, "command"="MEAS.requestAC", "command data"=w6926) -> (w6946:T11)
        n3142 = Bundle By Name(cluster=w6932, "command"="Apps.WaitForEvent", "command data"=w6926) -> (w6931:T11)
        n3143 = Bundle By Name(cluster=w6932, "command"="MEAS.DMM dual read") -> (w6947:T11)
        n3144 = Bundle By Name(cluster=w6932, "command"="Apps.UI Update 1") -> (w6933:T11)
        n3145 = Build Array(w6947, w6946, w6931, w6933) -> (w6944:T11[])
        n3146 = Build Array (concatenate)(w6945, w6944) -> (w6943:T11[])
        n3147 = for {
          tunnel: w6943 -> [w6980] mode=indexing
          tunnel: w6938 -> [w6981]
          tunnel: [w6977] -> w6941 mode=indexing
          n3148 = Unbundle By Name(w6980) -> ("command"=w6979:string, "command data"=w6978:variant)
          n3149 = call "App enquece.vi"("command data"=w6978, "command"=w6979, "queue in"=w6981) -> ("error out"=w6977:errorcluster)  [unwired: 7 in, 1 out]
        }
        n3150 = Merge Errors(w6942, w6941) -> (w6940:errorcluster)
      }
      frame "Test DRV 17A" {
        w6989 = T11 {"command"="", "command data"=variant} ("element")
        w6983 = 17 ("DUT index(0-59)")
        w7015 = T11 {"command"="", "command data"=variant} ("element")
        n3151 = disable-structure shown="LOGGING==TRUE" {
          disable-tunnel: w6993 -> [w7030 _]
          frame condition #0 (active) {
            n3152 = Empty String/Path?(string/path=w7030) -> (empty?=w7033:bool)
            n3153 = Select(t="Quece timeout", s=w7033, f=w7030) -> (s? t:f=w7029:string)
            n3154 = call "string log (SubVI).vi"("Enum"=enum16{"Init", "Log", "Read"}."Log", "state Name"=w7029) -> ()  [unwired: 8 in, 2 out]
          }
          frame condition #1 {
          }
        }
        n3155 = Flush Queue(queue=w6994) -> (queue out=w6995:refnum<queue>)  [unwired: 1 in, 2 out]
        n3156 = Decrement(x=w6983) -> (x-1=w6986:i32)
        n3157 = Index Array(array=w6982, index=w6986) -> (element=w6984:refnum<vi>)
        n3158 = property class="ColBox"(reference=w6984, "Value"=u32 10000536 ("DRV 1")) -> ()  [unwired: 1 in, 2 out]
        n3159 = To Variant(anything=bool[] [FALSE, FALSE, FALSE, FALSE, TRUE, FALSE]) -> (Variant=w7012:variant)
        n3160 = To Variant(anything=T6."demux1_10_channel3" ("demux1_10(x6)_encode")) -> (Variant=w7016:variant)
        n3161 = To Variant(anything=T4."mux6_1_channel5_3" ("mux6_1(3wires)_encode")) -> (Variant=w7019:variant)
        n3162 = To Variant(anything=T5."mux10_1_channel3" ("mux10_1(x6)_encode")) -> (Variant=w7021:variant)
        n3163 = Bundle By Name(cluster=w7015, "command"="MEAS.mux10-1", "command data"=w7021) -> (w7010:T11)
        n3164 = Bundle By Name(cluster=w7015, "command"="MEAS.mux6_1", "command data"=w7019) -> (w7009:T11)
        n3165 = Bundle By Name(cluster=w7015, "command"="MEAS.demux1-10", "command data"=w7016) -> (w7008:T11)
        n3166 = Bundle By Name(cluster=w7015, "command"="MEAS.eMIC", "command data"=w7012) -> (w7007:T11)
        n3167 = Bundle By Name(cluster=w7015, "command"="MEAS.AllRelaysOFF") -> (w7011:T11)
        n3168 = Build Array(w7011, w7010, w7009, w7008, w7007) -> (w7002:T11[])
        n3169 = Bundle By Name(cluster=w6989, "command"="Apps.WaitForEvent", "command data"=w6983) -> (w6988:T11)
        n3170 = Bundle By Name(cluster=w6989, "command"="MEAS.requestAC", "command data"=w6983) -> (w7003:T11)
        n3171 = Bundle By Name(cluster=w6989, "command"="Apps.UI Update 1") -> (w6990:T11)
        n3172 = Bundle By Name(cluster=w6989, "command"="MEAS.DMM dual read") -> (w7004:T11)
        n3173 = Build Array(w7004, w7003, w6988, w6990) -> (w7001:T11[])
        n3174 = Build Array (concatenate)(w7002, w7001) -> (w7000:T11[])
        n3175 = for {
          tunnel: w7000 -> [w7037] mode=indexing
          tunnel: w6995 -> [w7038]
          tunnel: [w7034] -> w6998 mode=indexing
          n3176 = Unbundle By Name(w7037) -> ("command"=w7036:string, "command data"=w7035:variant)
          n3177 = call "App enquece.vi"("command data"=w7035, "command"=w7036, "queue in"=w7038) -> ("error out"=w7034:errorcluster)  [unwired: 7 in, 1 out]
        }
        n3178 = Merge Errors(w6999, w6998) -> (w6997:errorcluster)
      }
      frame "Test DRV 18A" {
        w7046 = T11 {"command"="", "command data"=variant} ("element")
        w7040 = 18 ("DUT index(0-59)")
        w7072 = T11 {"command"="", "command data"=variant} ("element")
        n3179 = disable-structure shown="LOGGING==TRUE" {
          disable-tunnel: w7050 -> [w7087 _]
          frame condition #0 (active) {
            n3180 = Empty String/Path?(string/path=w7087) -> (empty?=w7090:bool)
            n3181 = Select(t="Quece timeout", s=w7090, f=w7087) -> (s? t:f=w7086:string)
            n3182 = call "string log (SubVI).vi"("Enum"=enum16{"Init", "Log", "Read"}."Log", "state Name"=w7086) -> ()  [unwired: 8 in, 2 out]
          }
          frame condition #1 {
          }
        }
        n3183 = Flush Queue(queue=w7051) -> (queue out=w7052:refnum<queue>)  [unwired: 1 in, 2 out]
        n3184 = Decrement(x=w7040) -> (x-1=w7043:i32)
        n3185 = Index Array(array=w7039, index=w7043) -> (element=w7041:refnum<vi>)
        n3186 = property class="ColBox"(reference=w7041, "Value"=u32 10000536 ("DRV 1")) -> ()  [unwired: 1 in, 2 out]
        n3187 = To Variant(anything=bool[] [FALSE, FALSE, FALSE, FALSE, FALSE, TRUE]) -> (Variant=w7069:variant)
        n3188 = To Variant(anything=T6."demux1_10_channel3" ("demux1_10(x6)_encode")) -> (Variant=w7073:variant)
        n3189 = To Variant(anything=T4."mux6_1_channel6_3" ("mux6_1(3wires)_encode")) -> (Variant=w7076:variant)
        n3190 = To Variant(anything=T5."mux10_1_channel3" ("mux10_1(x6)_encode")) -> (Variant=w7078:variant)
        n3191 = Bundle By Name(cluster=w7072, "command"="MEAS.mux10-1", "command data"=w7078) -> (w7067:T11)
        n3192 = Bundle By Name(cluster=w7072, "command"="MEAS.mux6_1", "command data"=w7076) -> (w7066:T11)
        n3193 = Bundle By Name(cluster=w7072, "command"="MEAS.demux1-10", "command data"=w7073) -> (w7065:T11)
        n3194 = Bundle By Name(cluster=w7072, "command"="MEAS.eMIC", "command data"=w7069) -> (w7064:T11)
        n3195 = Bundle By Name(cluster=w7072, "command"="MEAS.AllRelaysOFF") -> (w7068:T11)
        n3196 = Build Array(w7068, w7067, w7066, w7065, w7064) -> (w7059:T11[])
        n3197 = Bundle By Name(cluster=w7046, "command"="MEAS.requestAC", "command data"=w7040) -> (w7060:T11)
        n3198 = Bundle By Name(cluster=w7046, "command"="Apps.WaitForEvent", "command data"=w7040) -> (w7045:T11)
        n3199 = Bundle By Name(cluster=w7046, "command"="MEAS.DMM dual read") -> (w7061:T11)
        n3200 = Bundle By Name(cluster=w7046, "command"="Apps.UI Update 1") -> (w7047:T11)
        n3201 = Build Array(w7061, w7060, w7045, w7047) -> (w7058:T11[])
        n3202 = Build Array (concatenate)(w7059, w7058) -> (w7057:T11[])
        n3203 = for {
          tunnel: w7057 -> [w7094] mode=indexing
          tunnel: w7052 -> [w7095]
          tunnel: [w7091] -> w7055 mode=indexing
          n3204 = Unbundle By Name(w7094) -> ("command"=w7093:string, "command data"=w7092:variant)
          n3205 = call "App enquece.vi"("command data"=w7092, "command"=w7093, "queue in"=w7095) -> ("error out"=w7091:errorcluster)  [unwired: 7 in, 1 out]
        }
        n3206 = Merge Errors(w7056, w7055) -> (w7054:errorcluster)
      }
      frame "Test DRV 19A" {
        w7103 = T11 {"command"="", "command data"=variant} ("element")
        w7097 = 19 ("DUT index(0-59)")
        w7129 = T11 {"command"="", "command data"=variant} ("element")
        n3207 = disable-structure shown="LOGGING==TRUE" {
          disable-tunnel: w7107 -> [w7144 _]
          frame condition #0 (active) {
            n3208 = Empty String/Path?(string/path=w7144) -> (empty?=w7147:bool)
            n3209 = Select(t="Quece timeout", s=w7147, f=w7144) -> (s? t:f=w7143:string)
            n3210 = call "string log (SubVI).vi"("Enum"=enum16{"Init", "Log", "Read"}."Log", "state Name"=w7143) -> ()  [unwired: 8 in, 2 out]
          }
          frame condition #1 {
          }
        }
        n3211 = Flush Queue(queue=w7108) -> (queue out=w7109:refnum<queue>)  [unwired: 1 in, 2 out]
        n3212 = Decrement(x=w7097) -> (x-1=w7100:i32)
        n3213 = Index Array(array=w7096, index=w7100) -> (element=w7098:refnum<vi>)
        n3214 = property class="ColBox"(reference=w7098, "Value"=u32 10000536 ("DRV 1")) -> ()  [unwired: 1 in, 2 out]
        n3215 = To Variant(anything=bool[] [TRUE, FALSE, FALSE, FALSE, FALSE, FALSE]) -> (Variant=w7126:variant)
        n3216 = To Variant(anything=T6."demux1_10_channel4" ("demux1_10(x6)_encode")) -> (Variant=w7130:variant)
        n3217 = To Variant(anything=T4."mux6_1_channel1_3" ("mux6_1(3wires)_encode")) -> (Variant=w7133:variant)
        n3218 = To Variant(anything=T5."mux10_1_channel4" ("mux10_1(x6)_encode")) -> (Variant=w7135:variant)
        n3219 = Bundle By Name(cluster=w7129, "command"="MEAS.mux10-1", "command data"=w7135) -> (w7124:T11)
        n3220 = Bundle By Name(cluster=w7129, "command"="MEAS.mux6_1", "command data"=w7133) -> (w7123:T11)
        n3221 = Bundle By Name(cluster=w7129, "command"="MEAS.demux1-10", "command data"=w7130) -> (w7122:T11)
        n3222 = Bundle By Name(cluster=w7129, "command"="MEAS.eMIC", "command data"=w7126) -> (w7121:T11)
        n3223 = Bundle By Name(cluster=w7129, "command"="MEAS.AllRelaysOFF") -> (w7125:T11)
        n3224 = Build Array(w7125, w7124, w7123, w7122, w7121) -> (w7116:T11[])
        n3225 = Bundle By Name(cluster=w7103, "command"="MEAS.requestAC", "command data"=w7097) -> (w7117:T11)
        n3226 = Bundle By Name(cluster=w7103, "command"="Apps.WaitForEvent", "command data"=w7097) -> (w7102:T11)
        n3227 = Bundle By Name(cluster=w7103, "command"="MEAS.DMM dual read") -> (w7118:T11)
        n3228 = Bundle By Name(cluster=w7103, "command"="Apps.UI Update 1") -> (w7104:T11)
        n3229 = Build Array(w7118, w7117, w7102, w7104) -> (w7115:T11[])
        n3230 = Build Array (concatenate)(w7116, w7115) -> (w7114:T11[])
        n3231 = for {
          tunnel: w7114 -> [w7151] mode=indexing
          tunnel: w7109 -> [w7152]
          tunnel: [w7148] -> w7112 mode=indexing
          n3232 = Unbundle By Name(w7151) -> ("command"=w7150:string, "command data"=w7149:variant)
          n3233 = call "App enquece.vi"("command data"=w7149, "command"=w7150, "queue in"=w7152) -> ("error out"=w7148:errorcluster)  [unwired: 7 in, 1 out]
        }
        n3234 = Merge Errors(w7113, w7112) -> (w7111:errorcluster)
      }
      frame "Test DRV 20A" {
        w7160 = T11 {"command"="", "command data"=variant} ("element")
        w7154 = 20 ("DUT index(0-59)")
        w7186 = T11 {"command"="", "command data"=variant} ("element")
        n3235 = disable-structure shown="LOGGING==TRUE" {
          disable-tunnel: w7164 -> [w7201 _]
          frame condition #0 (active) {
            n3236 = Empty String/Path?(string/path=w7201) -> (empty?=w7204:bool)
            n3237 = Select(t="Quece timeout", s=w7204, f=w7201) -> (s? t:f=w7200:string)
            n3238 = call "string log (SubVI).vi"("Enum"=enum16{"Init", "Log", "Read"}."Log", "state Name"=w7200) -> ()  [unwired: 8 in, 2 out]
          }
          frame condition #1 {
          }
        }
        n3239 = Flush Queue(queue=w7165) -> (queue out=w7166:refnum<queue>)  [unwired: 1 in, 2 out]
        n3240 = Decrement(x=w7154) -> (x-1=w7157:i32)
        n3241 = Index Array(array=w7153, index=w7157) -> (element=w7155:refnum<vi>)
        n3242 = property class="ColBox"(reference=w7155, "Value"=u32 10000536 ("DRV 1")) -> ()  [unwired: 1 in, 2 out]
        n3243 = To Variant(anything=bool[] [FALSE, TRUE, FALSE, FALSE, FALSE, FALSE]) -> (Variant=w7183:variant)
        n3244 = To Variant(anything=T6."demux1_10_channel4" ("demux1_10(x6)_encode")) -> (Variant=w7187:variant)
        n3245 = To Variant(anything=T4."mux6_1_channel2_3" ("mux6_1(3wires)_encode")) -> (Variant=w7190:variant)
        n3246 = To Variant(anything=T5."mux10_1_channel4" ("mux10_1(x6)_encode")) -> (Variant=w7192:variant)
        n3247 = Bundle By Name(cluster=w7186, "command"="MEAS.mux10-1", "command data"=w7192) -> (w7181:T11)
        n3248 = Bundle By Name(cluster=w7186, "command"="MEAS.mux6_1", "command data"=w7190) -> (w7180:T11)
        n3249 = Bundle By Name(cluster=w7186, "command"="MEAS.demux1-10", "command data"=w7187) -> (w7179:T11)
        n3250 = Bundle By Name(cluster=w7186, "command"="MEAS.eMIC", "command data"=w7183) -> (w7178:T11)
        n3251 = Bundle By Name(cluster=w7186, "command"="MEAS.AllRelaysOFF") -> (w7182:T11)
        n3252 = Build Array(w7182, w7181, w7180, w7179, w7178) -> (w7173:T11[])
        n3253 = Bundle By Name(cluster=w7160, "command"="MEAS.requestAC", "command data"=w7154) -> (w7174:T11)
        n3254 = Bundle By Name(cluster=w7160, "command"="Apps.WaitForEvent", "command data"=w7154) -> (w7159:T11)
        n3255 = Bundle By Name(cluster=w7160, "command"="MEAS.DMM dual read") -> (w7175:T11)
        n3256 = Bundle By Name(cluster=w7160, "command"="Apps.UI Update 1") -> (w7161:T11)
        n3257 = Build Array(w7175, w7174, w7159, w7161) -> (w7172:T11[])
        n3258 = Build Array (concatenate)(w7173, w7172) -> (w7171:T11[])
        n3259 = for {
          tunnel: w7171 -> [w7208] mode=indexing
          tunnel: w7166 -> [w7209]
          tunnel: [w7205] -> w7169 mode=indexing
          n3260 = Unbundle By Name(w7208) -> ("command"=w7207:string, "command data"=w7206:variant)
          n3261 = call "App enquece.vi"("command data"=w7206, "command"=w7207, "queue in"=w7209) -> ("error out"=w7205:errorcluster)  [unwired: 7 in, 1 out]
        }
        n3262 = Merge Errors(w7170, w7169) -> (w7168:errorcluster)
      }
      frame "Test DRV 21A" {
        w7217 = T11 {"command"="", "command data"=variant} ("element")
        w7210 = 21 ("DUT index(0-59)")
        w7243 = T11 {"command"="", "command data"=variant} ("element")
        n3263 = disable-structure shown="LOGGING==TRUE" {
          disable-tunnel: w7221 -> [w7258 _]
          frame condition #0 (active) {
            n3264 = Empty String/Path?(string/path=w7258) -> (empty?=w7261:bool)
            n3265 = Select(t="Quece timeout", s=w7261, f=w7258) -> (s? t:f=w7257:string)
            n3266 = call "string log (SubVI).vi"("Enum"=enum16{"Init", "Log", "Read"}."Log", "state Name"=w7257) -> ()  [unwired: 8 in, 2 out]
          }
          frame condition #1 {
          }
        }
        n3267 = Flush Queue(queue=w7222) -> (queue out=w7223:refnum<queue>)  [unwired: 1 in, 2 out]
        n3268 = Decrement(x=w7210) -> (x-1=w7214:i32)
        n3269 = Index Array(array=w7211, index=w7214) -> (element=w7212:refnum<vi>)
        n3270 = property class="ColBox"(reference=w7212, "Value"=u32 10000536 ("DRV 1")) -> ()  [unwired: 1 in, 2 out]
        n3271 = To Variant(anything=bool[] [FALSE, FALSE, TRUE, FALSE, FALSE, FALSE]) -> (Variant=w7240:variant)
        n3272 = To Variant(anything=T6."demux1_10_channel4" ("demux1_10(x6)_encode")) -> (Variant=w7244:variant)
        n3273 = To Variant(anything=T4."mux6_1_channel3_3" ("mux6_1(3wires)_encode")) -> (Variant=w7247:variant)
        n3274 = To Variant(anything=T5."mux10_1_channel4" ("mux10_1(x6)_encode")) -> (Variant=w7249:variant)
        n3275 = Bundle By Name(cluster=w7243, "command"="MEAS.mux10-1", "command data"=w7249) -> (w7238:T11)
        n3276 = Bundle By Name(cluster=w7243, "command"="MEAS.mux6_1", "command data"=w7247) -> (w7237:T11)
        n3277 = Bundle By Name(cluster=w7243, "command"="MEAS.demux1-10", "command data"=w7244) -> (w7236:T11)
        n3278 = Bundle By Name(cluster=w7243, "command"="MEAS.eMIC", "command data"=w7240) -> (w7235:T11)
        n3279 = Bundle By Name(cluster=w7243, "command"="MEAS.AllRelaysOFF") -> (w7239:T11)
        n3280 = Build Array(w7239, w7238, w7237, w7236, w7235) -> (w7230:T11[])
        n3281 = Bundle By Name(cluster=w7217, "command"="MEAS.requestAC", "command data"=w7210) -> (w7231:T11)
        n3282 = Bundle By Name(cluster=w7217, "command"="Apps.WaitForEvent", "command data"=w7210) -> (w7216:T11)
        n3283 = Bundle By Name(cluster=w7217, "command"="MEAS.DMM dual read") -> (w7232:T11)
        n3284 = Bundle By Name(cluster=w7217, "command"="Apps.UI Update 1") -> (w7218:T11)
        n3285 = Build Array(w7232, w7231, w7216, w7218) -> (w7229:T11[])
        n3286 = Build Array (concatenate)(w7230, w7229) -> (w7228:T11[])
        n3287 = for {
          tunnel: w7228 -> [w7265] mode=indexing
          tunnel: w7223 -> [w7266]
          tunnel: [w7262] -> w7226 mode=indexing
          n3288 = Unbundle By Name(w7265) -> ("command"=w7264:string, "command data"=w7263:variant)
          n3289 = call "App enquece.vi"("command data"=w7263, "command"=w7264, "queue in"=w7266) -> ("error out"=w7262:errorcluster)  [unwired: 7 in, 1 out]
        }
